vi "test_ParseSolutionFile_DifferentPathFormats.vi"() -> (3 "Pass?":bool)   [LabVIEW 2019, in "Tests.SolutionBuilder.lvlib"]
uses:
  Tests.SolutionBuilder.lvlib
  SolutionBuilder/SolutionBuilder.lvclass
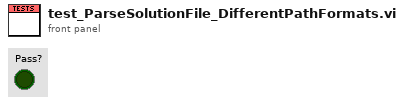
[diagram p1: front panel]
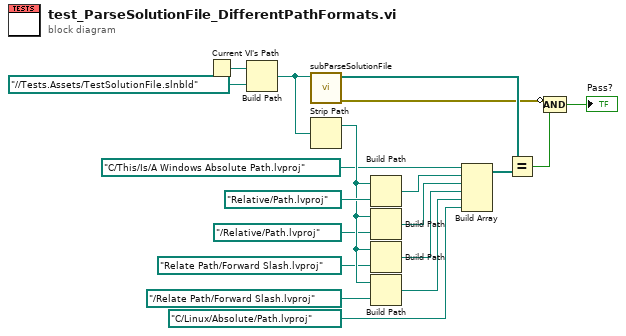
[diagram p0: block diagram]
diagram:
  n1 = Current VI's Path() -> (path=w18:path)
  n2 = Build Path(base path=w18, name or relative path=path "../../Tests.Assets/TestSolutionFile.slnbld" ("Path")) -> (appended path=w4:path)
  n3 = call "subParseSolutionFile.vi"("Solution file"=w4) -> ("error out"=w2:errorcluster, "Projects"=w3:path[])  [unwired: 7 in, 2 out]
  n4 = Strip Path(path=w4) -> (stripped path=w15:path)  [unwired: 1 out]
  n5 = Build Path(base path=w15, name or relative path=path "Relative/Path.lvproj" ("Path")) -> (appended path=w10:path)
  n6 = Build Path(base path=w15, name or relative path=path "../Relative/Path.lvproj" ("Path")) -> (appended path=w9:path)
  n7 = Build Path(base path=w15, name or relative path=path "Relate Path/Forward Slash.lvproj" ("Path")) -> (appended path=w8:path)
  n8 = Build Path(base path=w15, name or relative path=path "../Relate Path/Forward Slash.lvproj" ("Path")) -> (appended path=w7:path)
  n9 = Build Array(path "C:/This/Is/A Windows Absolute Path.lvproj" ("Path"), w10, w9, w8, w7, path "C:/Linux/Absolute/Path.lvproj" ("Path")) -> (w5:path[])
  n10 = Equal?(x=w3, y=w5) -> (x = y?=w1:bool)
  n11 = Compound Arithmetic op=AND(invert w2, w1) -> (→"Pass?":bool)
